vi "INIT swerve.vi"(8 "error in (no error)":errorcluster) -> (0 "error out":errorcluster)   [LabVIEW 2023]
uses:
  <vilib>/Rock Robotics/WPI/ThirdParty/REV Robotics/REVLib/Typedef/Spark MAX Sensor Type.ctl
  <vilib>/Rock Robotics/WPI/ThirdParty/REV Robotics/REVLib/Typedef/Spark MAX Control Type.ctl
  Global INIT.vi
panel:
  out "x/y 2":dbl
  out "x/y":dbl
  in  "DRIVE RAMP":sgl=0.05
  out "deg/tic":dbl
  out "STEER deg/motor rev":dbl=16.800001120000072
  out "DRIVE in/motor rev":dbl=0.1551403779550515
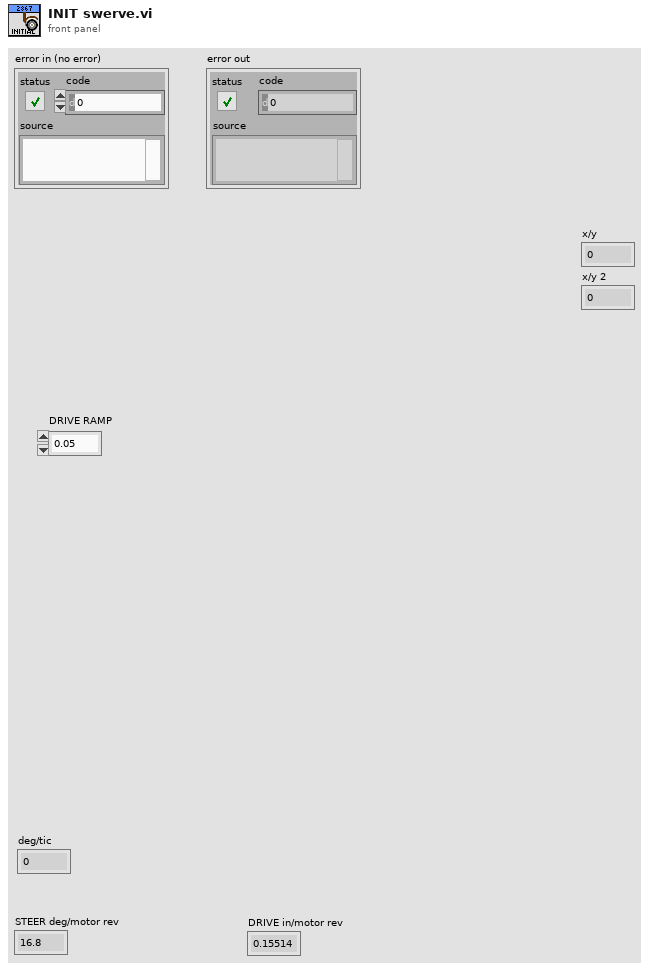
[diagram p1: front panel]
types:
  T1 = typedef "ctrl robot swerve dims.ctl" = cluster{"drive track":dbl, "drive base":dbl, "wheel  (in)":dbl, "steer ratio":dbl, "drive ratio":dbl, "enc ratio":dbl}
  T2 = typedef "ctrl swerve motor.ctl" = cluster{"description":string, "MOTOR SELECT":T3, "Installed?":bool, "CAN ID":u8, "refnum name":string, "Invert":bool, "Idle Mode":T4, "Current limiting":T5, "MOTOR PIDF coefficients":T6, "gear ratio":dbl}
  T3 = typedef "ctrl MOTOR SELECT.ctl" = i16
  T4 = typedef "Spark MAX Idle Mode.ctl" = enum16{"Coast", "Brake"}
  T5 = typedef "ctrl Spark MAX current limiting.ctl" = cluster{"Linearized":bool, "Free Speed (A)":dbl, "Primay (A)":dbl, "Limit RPM (0)":u32}
  T6 = typedef "ctrl motor PIDF coefficients.ctl" = cluster{"PIDF":cluster{"P Gain":dbl, "I Gain":dbl, "D Gain":dbl, "F Gain":dbl, "I Zone":dbl, "Min Output":dbl, "Max Output":dbl}, "Smart Motion":T7}
  T7 = typedef "Spark MAX Smart Motion Parameters.ctl" = cluster{"Max Velocity":dbl, "Max Acceleration":dbl, "Minimum Velocity Output":dbl, "Allowed Closed Loop Error":dbl}
  T8 = typedef "ctrl CANcoder.ctl" = cluster{"description":string, "Installed?":bool, "CAN ID":u8, "CAN Bus":string, "refnum name":string, "Sensor Direction":bool, "Magnet Offset (Degrees)":dbl}
  T9 = typedef "Spark MAX Control Type.ctl" = enum16{"Percent VBus", "Voltage", "Velocity", "Position", "Smart Motion", "Current", "Smart Velocity"}
  T10 = typedef "Spark MAX Sensor Type.ctl" = enum16{"No Sensor", "Hall Sensor", "Encoder", "-Not Available-", "Analog", "Alternate Encoder", "Duty Cycle"}
  T11 = typedef "WPI_MotorControlDeviceRef.ctl" = cluster{"DeviceStatus":errorcluster, "Type":T12, "PWM":cluster{"PWM Channel":T13, "DeadBand":T14}, "CAN":cluster{"Device Number":u8, "SetOutput VI Ref":variant, "GetOutput VI Ref":variant, "Enable VI Ref":variant, "Disable VI Ref":variant, "Data":variant}, "Invert":bool, "DIO PWM":cluster{"PWM \"Enable\" Channel":T13, "DIOChannel":T15, "PWM Rate":dbl}}
  T12 = typedef "WPI_MotorControlType.ctl" = enum16{"PWM", "CAN", "DIO PWM"}
  T13 = typedef "FPGA_DIOPWMChannel.ctl" = enum8{"PWM 0", "PWM 1", "PWM 2", "PWM 3", "PWM 4", "PWM 5", "PWM 6", "PWM 7", "PWM 8", "PWM 9", "PWM MXP 0", "PWM MXP 1", "PWM MXP 2", "PWM MXP 3", "PWM MXP 4", "PWM MXP 5", "PWM MXP 6", "PWM MXP 7", "PWM MXP 8", "PWM MXP 9", "Invalid"}
  T14 = typedef "WPI_PWMDeadband.ctl" = cluster{"Name":string, "maxPositivePwm":i32, "minPositivePwm":i32, "centerPwm":i32, "maxNegativePwm":i32, "minNegativePwm":i32, "angularRange":u16}
  T15 = typedef "FPGA_DIOChannel.ctl" = enum8{"DIO 0", "DIO 1", "DIO 2", "DIO 3", "DIO 4", "DIO 5", "DIO 6", "DIO 7", "DIO 8", "DIO 9", "DIO MXP 0", "DIO MXP 1", "DIO MXP 2", "DIO MXP 3", "DIO MXP 4", "DIO MXP 5", "DIO MXP 6", "DIO MXP 7", "DIO MXP 8", "DIO MXP 9", "DIO MXP 10", "DIO MXP 11", "DIO MXP 12", "DIO MXP 13", "DIO MXP 14", "DIO MXP 15", "SPI Port CS1", "SPI Port CS2", "SPI Port CS3", "SPI Port MISO", "SPI Port MOSI", "Invalid"}
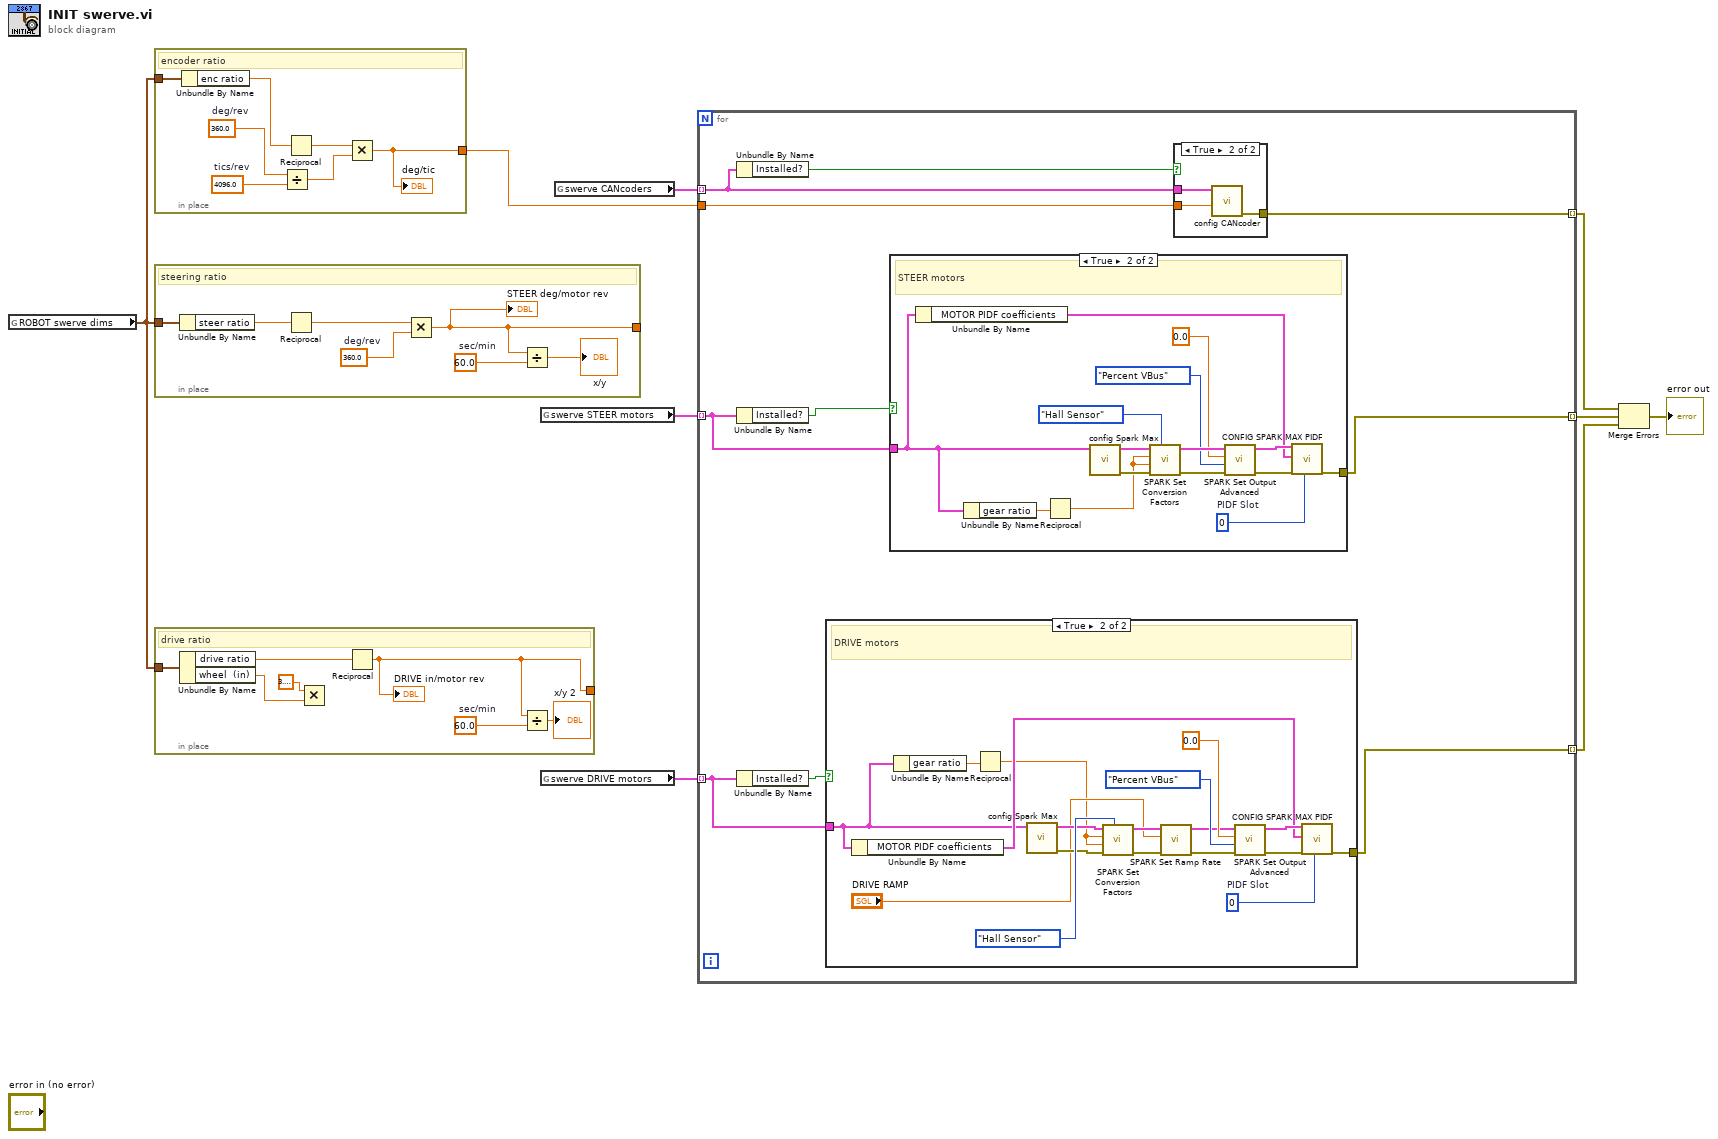
[diagram p0: block diagram]
diagram:
  n1 = global read "Global INIT.vi" "ROBOT swerve dims"() -> (w5:T1)
  n2 = in-place {
    in-place-border: w5 -> [w16]
    in-place-border: [w10] -> w6
    w12 = 4096.0  # tics/rev
    w13 = 360.0  # deg/rev
    # "encoder ratio"
    n3 = Unbundle By Name(w16) -> ("enc ratio"=w15:dbl)
    n4 = Divide(x=w13, y=w12) -> (x/y=w11:dbl)
    n5 = Reciprocal(x=w15) -> (1/x=w14:dbl)
    n6 = Multiply(x=w14, y=w11) -> (x*y=w10:dbl)
    "deg/tic" <- w10
  }
  n7 = in-place {
    in-place-border: w5 -> [w19]
    in-place-border: [w18] -> _
    w21 = 60.0  # sec/min
    w22 = 360.0  # deg/rev
    # "steering ratio"
    n8 = Unbundle By Name(w19) -> ("steer ratio"=w20:dbl)
    n9 = Reciprocal(x=w20) -> (1/x=w23:dbl)
    n10 = Multiply(x=w23, y=w22) -> (x*y=w18:dbl)
    "STEER deg/motor rev" <- w18
    n11 = Divide(x=w18, y=w21) -> (x/y=→"x/y":dbl)
  }
  n12 = in-place {
    in-place-border: w5 -> [w27]
    in-place-border: [w30] -> _
    w28 = 60.0  # sec/min
    # "drive ratio"
    n13 = Unbundle By Name(w27) -> ("drive ratio"=w26:dbl, "wheel  (in)"=w25:dbl)
    n14 = Multiply(x=3.141592653589793, y=w25) -> ()  [unwired: 1 out]
    n15 = Reciprocal(x=w26) -> (1/x=w30:dbl)
    "DRIVE in/motor rev" <- w30
    n16 = Divide(x=w30, y=w28) -> (x/y=→"x/y 2":dbl)
  }
  n17 = global read "Global INIT.vi" "swerve STEER motors"() -> (w7:T2[])
  n18 = global read "Global INIT.vi" "swerve DRIVE motors"() -> (w9:T2[])
  n19 = global read "Global INIT.vi" "swerve CANcoders"() -> (w8:T8[])
  n20 = for {
    tunnel: w7 -> [w38] mode=indexing
    tunnel: w8 -> [w36] mode=indexing
    tunnel: w9 -> [w39] mode=indexing
    tunnel: w6 -> [w34]
    tunnel: [w33] -> w3 mode=indexing
    tunnel: [w32] -> w2 mode=indexing
    tunnel: [w31] -> w4 mode=indexing
    n21 = Unbundle By Name(w36) -> ("Installed?"=w35:bool)
    n22 = Unbundle By Name(w38) -> ("Installed?"=w37:bool)
    n23 = Unbundle By Name(w39) -> ("Installed?"=w40:bool)
    n24 = case shown="True" w40 {
      tunnel: w39 -> [_ w59]
      tunnel: [_ w66] -> w32
      frame False {
      }
      frame True {
        w63 = 0  # PIDF Slot
        # "DRIVE motors"
        n25 = Unbundle By Name(w59) -> ("MOTOR PIDF coefficients"=w62:T6)
        n26 = Unbundle By Name(w59) -> ("gear ratio"=w61:dbl)
        n27 = Reciprocal(x=w61) -> (1/x=w60:dbl)
        n28 = call "config Spark Max.vi"("motor\ndefaults"=w59) -> ("error out"=w72:errorcluster, "MotorControlDevRef"=w73:T11)  [unwired: 9 in]
        n29 = call <vilib>:"SPARK Set Conversion Factors.vi"("Sensor Type (Hall Sensor)"=Spark_MAX_Sensor_Type."Hall Sensor", "error in (no error)"=w72, "Velocity Factor (1)"=w60, "Position Factor (1)"=w60, "MotorControlDeviceRef in"=w73) -> ("error out"=w68:errorcluster, "MotorControlDeviceRef out"=w75:T11)  [unwired: 5 in]
        n30 = call <vilib>:"SPARK Set Ramp Rate.vi"("error in (no error)"=w68, "Seconds from neutral to full (0)"="DRIVE RAMP", "MotorControlDeviceRef in"=w75) -> ("error out"=w67:errorcluster, "MotorControlDeviceRef"=w70:T11)  [unwired: 7 in]
        n31 = call <vilib>:"SPARK Set Output Advanced.vi"("error in (no error)"=w67, "Control Mode"=Spark_MAX_Control_Type."Percent VBus", "Setpoint"=0.0 ("Output"), "MotorControlDevRef"=w70) -> ("error out"=w64:errorcluster, "MotorControlDevRef"=w65:T11)  [unwired: 6 in]
        n32 = call "CONFIG SPARK MAX PIDF.vi"("MotorControlDevRef"=w65, "MOTOR PIDF coefficients"=w62, "error in (no error)"=w64, "PIDF Slot"=w63) -> ("error out"=w66:errorcluster)  [unwired: 14 in, 1 out]
      }
    }
    n33 = case shown="True" w37 {
      tunnel: w38 -> [_ w44]
      tunnel: [_ w50] -> w33
      frame False {
      }
      frame True {
        w49 = 0  # PIDF Slot
        # "STEER motors"
        n34 = Unbundle By Name(w44) -> ("MOTOR PIDF coefficients"=w47:T6)
        n35 = Unbundle By Name(w44) -> ("gear ratio"=w46:dbl)
        n36 = Reciprocal(x=w46) -> (1/x=w45:dbl)
        n37 = call "config Spark Max.vi"("motor\ndefaults"=w44) -> ("error out"=w53:errorcluster, "MotorControlDevRef"=w54:T11)  [unwired: 9 in]
        n38 = call <vilib>:"SPARK Set Conversion Factors.vi"("Sensor Type (Hall Sensor)"=Spark_MAX_Sensor_Type."Hall Sensor", "error in (no error)"=w53, "Velocity Factor (1)"=w45, "Position Factor (1)"=w45, "MotorControlDeviceRef in"=w54) -> ("error out"=w57:errorcluster, "MotorControlDeviceRef out"=w56:T11)  [unwired: 5 in]
        n39 = call <vilib>:"SPARK Set Output Advanced.vi"("error in (no error)"=w57, "Control Mode"=Spark_MAX_Control_Type."Percent VBus", "Setpoint"=0.0 ("Output"), "MotorControlDevRef"=w56) -> ("error out"=w51:errorcluster, "MotorControlDevRef"=w48:T11)  [unwired: 6 in]
        n40 = call "CONFIG SPARK MAX PIDF.vi"("MotorControlDevRef"=w48, "MOTOR PIDF coefficients"=w47, "error in (no error)"=w51, "PIDF Slot"=w49) -> ("error out"=w50:errorcluster)  [unwired: 14 in, 1 out]
      }
    }
    n41 = case shown="True" w35 {
      tunnel: w36 -> [_ w43]
      tunnel: w34 -> [_ w42]
      tunnel: [_ w41] -> w31
      frame False {
      }
      frame True {
        n42 = call "config CANcoder.vi"("SensorCoefficient"=w42, "CANcoder init data"=w43) -> ("error out"=w41:errorcluster)  [unwired: 9 in]
      }
    }
  }
  n43 = Merge Errors(w4, w3, w2) -> (→"error out":errorcluster)
